vi "Panel.vi"(11 "Team Field Panel in":refnum<class "Team Field Panel.lvclass">) -> ()   [LabVIEW 2020, in "SB App.lvlib" / "Team Field Panel.lvclass"]
uses:
  Team Field Panel.lvclass
  C:/Program Files (x86)/National Instruments/LabVIEW 2020/vi.lib/IlluminatedG/IG OOPanel/OOPanel/Panel/Panel.lvclass
  <vilib>/IlluminatedG/IG OOPanel/OOPanel/Panel/Basic UI State.ctl
  <vilib>/IlluminatedG/IG OOPanel/OOPanel/Panel/Panel.lvclass
  <vilib>/IlluminatedG/IG OOPanel/OOPanel/OOPanel.lvlib
  SquareBattle/SquareBattle.lvlib
panel:
  out "Team Field":i32[][](graph)
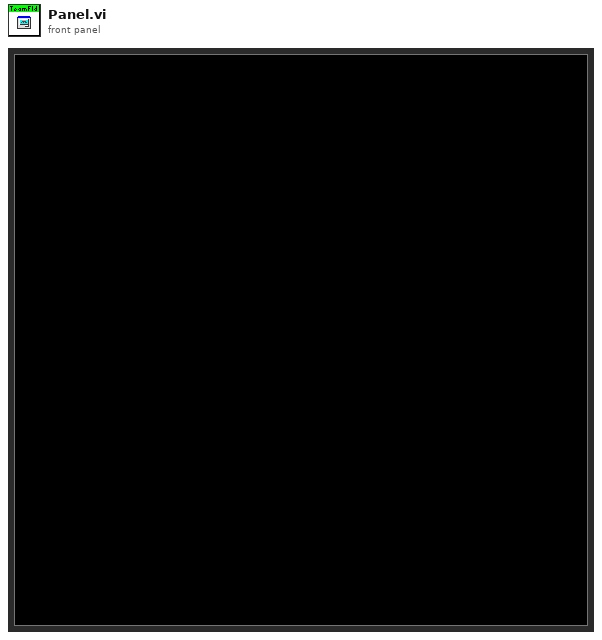
[diagram p1: front panel]
types:
  T1 = typedef "OOPanel.lvlib/Panel.lvclass/Basic UI State.ctl" = enum16{"Init", "Run", "Close"}
  T2 = typedef "OOPanel.lvlib/Panel.lvclass/Panel Events.ctl" = cluster{"Visbility":refnum<user-event>, "Close":refnum<user-event>}
  T3 = typedef "OOPanel.lvlib/Panel.lvclass/Visibility State.ctl" = enum16{"Idle", "Closed", "Hidden", "Visible", "Subpanel"}
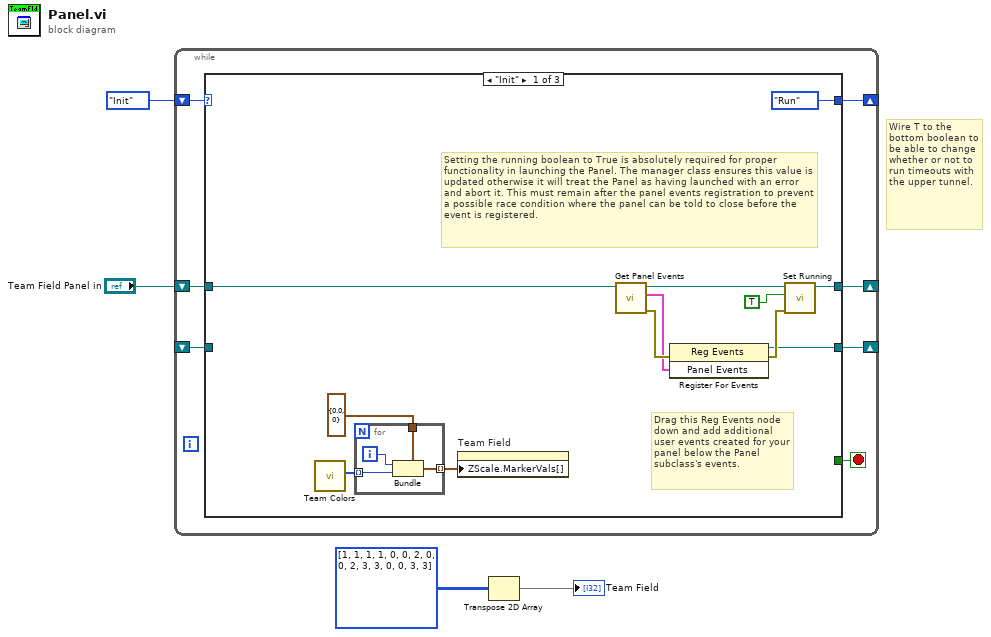
[diagram p0: block diagram]
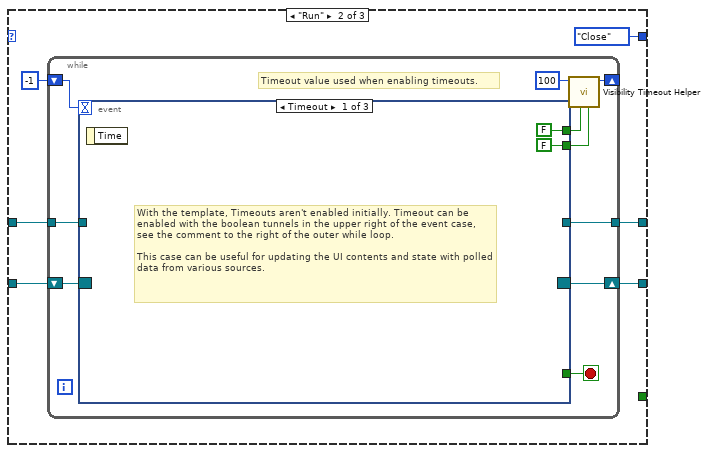
[diagram p2: hidden frame]
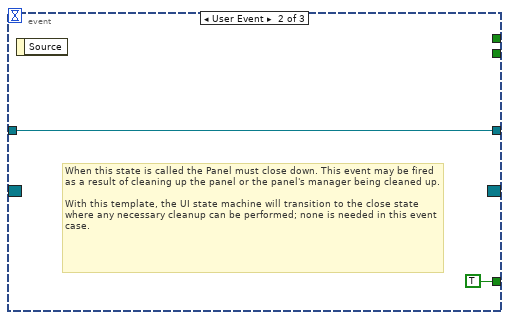
[diagram p3: hidden frame]
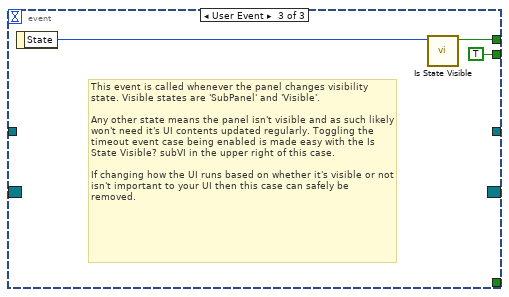
[diagram p4: hidden frame]
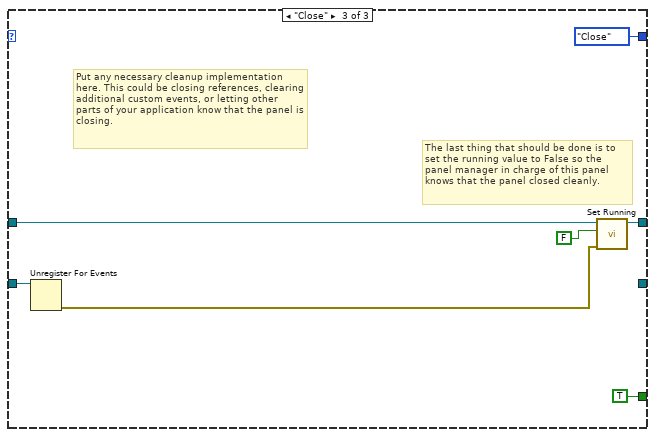
[diagram p5: hidden frame]
diagram:
  # "Wire T to the bottom boolean to be able to change whether or not to run timeouts with the upper tunnel."
  n1 = while {
    shift-right: [w10] -> _
    shift-left: _ -> [w11]
    shift-right: [w8] -> _
    shift-left: Basic_UI_State."Init" ("Basic UI State") -> [w9]
    shift-right: [w6] -> _
    shift-left: "Team Field Panel in" -> [w5]
    stop <- w7 stop-if-true
    n2 = case shown="\"Init\"" w9 {
      tunnel: w11 -> [_ w33 w53]
      tunnel: [w17 w31 _] -> w10
      tunnel: [Basic_UI_State."Run" ("Basic UI State") Basic_UI_State."Close" ("Basic UI State") Basic_UI_State."Close" ("Basic UI State")] -> w8
      tunnel: [_ _ TRUE] -> w7
      tunnel: [w16 w28 w51] -> w6
      tunnel: w5 -> [w15 w29 w52]
      frame "Init" {
        # "Setting the running boolean to True is absolutely required for proper functionality in launching the Panel. The manager class ensures this value is updated otherwise it will treat the Panel as having launched with an error and abort it. This must remain after the panel events registration to prevent a possible race condition where the panel can be told to close before the event is registered."
        # "Drag this Reg Events node down and add additional user events created for your panel below the Panel subclass's events."
        n3 = call "Team Colors.vi"() -> ("Team Colors"=w14:u32[])  [unwired: 11 in]
        n4 = for {
          tunnel: w14 -> [w27] mode=indexing
          tunnel: cluster{dbl, u32} {0.0, 0} -> [w26]
          tunnel: [w24] -> w12 mode=indexing
          i -> [w25]
          n5 = Bundle(cluster=w26, w25, w27) -> (w24:cluster{dbl, u32})
        }
        n6 = property on="Team Field" class="IntGraph (strict)"("ZScale.MarkerVals[]"=w12) -> ()  [unwired: 2 in, 2 out]
        n7 = call <vilib>:"Get Panel Events.vi"("Panel in"=w15) -> ("error out"=w23:errorcluster, "Panel Events"=w19:T2, "Panel out"=w20:refnum<class "Team Field Panel.lvclass">)  [unwired: 8 in]
        n8 = register-events(error in=w23, w19) -> (reference out=w17:refnum<event-registration>, error out=w21:errorcluster)  [unwired: 1 in]
        n9 = call <vilib>:"Set Running.vi"("error in (no error)"=w21, "Running"=TRUE, "Panel in"=w20) -> ("Panel out"=w16:refnum<class "Team Field Panel.lvclass">)  [unwired: 7 in, 1 out]
      }
      frame "Run" {
        n10 = while {
          shift-right: [w39] -> w31
          shift-left: w33 -> [w40]
          shift-right: [w42] -> _
          shift-left: -1 ("Timeout") -> [w41]
          tunnel: w29 -> [w35]
          tunnel: [w34] -> w28
          stop <- w36 stop-if-true
          # "Timeout value used when enabling timeouts."
          n11 = event shown="[0] Timeout" {
            selector: w40 -> [_ _ _]
            dyn-events: [_ _ _] -> w39
            timeout: w41 -> [_ _ _]
            tunnel: [FALSE _ w49] -> w38
            tunnel: [FALSE _ TRUE] -> w37
            tunnel: [_ TRUE _] -> w36
            tunnel: w35 -> [_ w46 _]
            tunnel: [_ w46 _] -> w34
            event Timeout {
              # "With the template, Timeouts aren't enabled initially. Timeout can be enabled with the boolean tunnels in the upper right of the event case, see the comment to the right of the outer while loop.\n\nThis case can be useful for updating the UI contents and state with polled data from various sources."
              n12 = event-data() -> ()  [unwired: 1 in, 1 out]
            }
            event User Event {
              # "When this state is called the Panel must close down. This event may be fired as a result of cleaning up the panel or the panel's manager being cleaned up.\n\nWith this template, the UI state machine will transition to the close state where any necessary cleanup can be performed; none is needed in this event case."
              n13 = event-data() -> ()  [unwired: 1 in, 1 out]
            }
            event User Event {
              # "This event is called whenever the panel changes visibility state. Visible states are 'SubPanel' and 'Visible'.\n\nAny other state means the panel isn't visible and as such likely won't need it's UI contents updated regularly. Toggling the timeout event case being enabled is made easy with the Is State Visible? subVI in the upper right of this case.\n\nIf changing how the UI runs based on whether it's visible or not isn't important to your UI then this case can safely be removed."
              n14 = event-data() -> ("State"=w50:T3)  [unwired: 1 in]
              n15 = call <vilib>:"Is State Visible.vi"("Visibility"=w50) -> ("Visible"=w49:bool)  [unwired: 10 in]
            }
          }
          n16 = call <vilib>:"Visibility Timeout Helper.vi"("Update?"=w37, "Use Timeout?"=w38, "Visible Timeout mS"=100) -> ("Timeout"=w42:i32)  [unwired: 8 in]
        }
      }
      frame "Close" {
        # "Put any necessary cleanup implementation here. This could be closing references, clearing additional custom events, or letting other parts of your application know that the panel is closing."
        # "The last thing that should be done is to set the running value to False so the panel manager in charge of this panel knows that the panel closed cleanly."
        n17 = Unregister For Events(event registration refnum=w53) -> (error out=w55:errorcluster)  [unwired: 1 in]
        n18 = call <vilib>:"Set Running.vi"("error in (no error)"=w55, "Running"=FALSE, "Panel in"=w52) -> ("Panel out"=w51:refnum<class "Team Field Panel.lvclass">)  [unwired: 7 in, 1 out]
      }
    }
  }
  n19 = Transpose 2D Array(2D array=i32[][] [[1, 1, 1, 1], [0, 0, 2, 0], [0, 2, 3, 3], [0, 0, 3, 3]] ("Team Field")) -> (transposed array=→"Team Field":i32[][])
